vi "ex_1_main.vi"() -> ()   [LabVIEW 2020]
uses:
  <vilib>/DAQmx/read.llb/DAQmx Read (Analog 1D Wfm NChan NSamp).vi
  <vilib>/DAQmx/create/channels.llb/DAQmx Create Channel (AI-Voltage-Basic).vi
  <vilib>/DAQmx/configure/timing.llb/DAQmx Timing (Sample Clock).vi
  <vilib>/DAQmx/configure/trigger.llb/DAQmx Start Trigger (Digital Edge).vi
  <vilib>/DAQmx/miscellaneous.llb/DAQmx Fill In Error Info.vi
panel:
  out "current time 2":timestamp
  out "current time":timestamp
  out "Numeric 2":dbl
  out "Numeric":i32
  out "Waveform Graph":waveform(dbl)[](graph)
  in  "stop":bool
  # "Pomiar ciągły z 3 kanałów dowolnej (np. 6259) karty pomiarowej symulowanej w MAX dla pomiaru sygnału o częstotliwości 15kHz. Pomiar rozpoczyna się po wystąpieniu triggera na linii PFI0 wybranej karty pomiarowej."
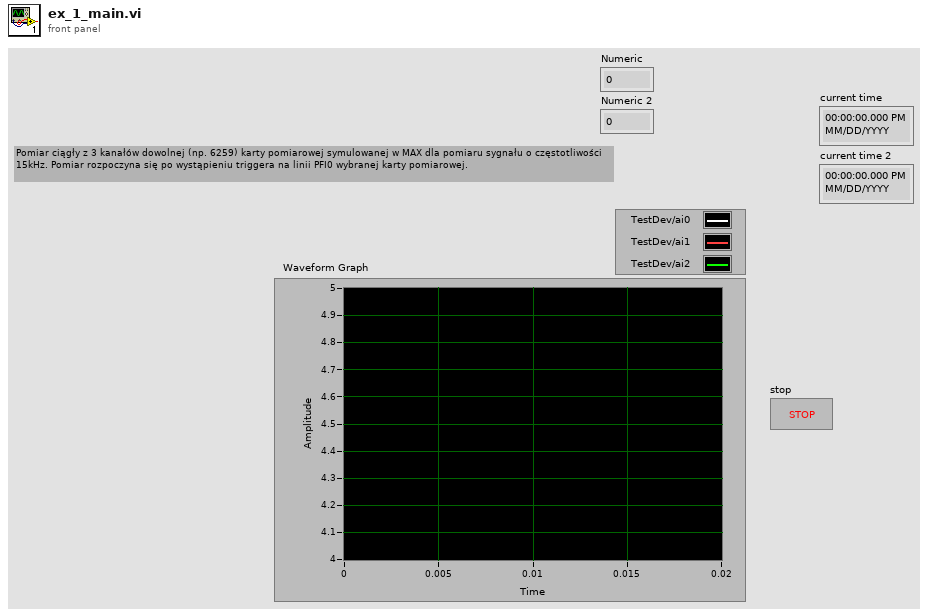
[diagram p1: front panel]
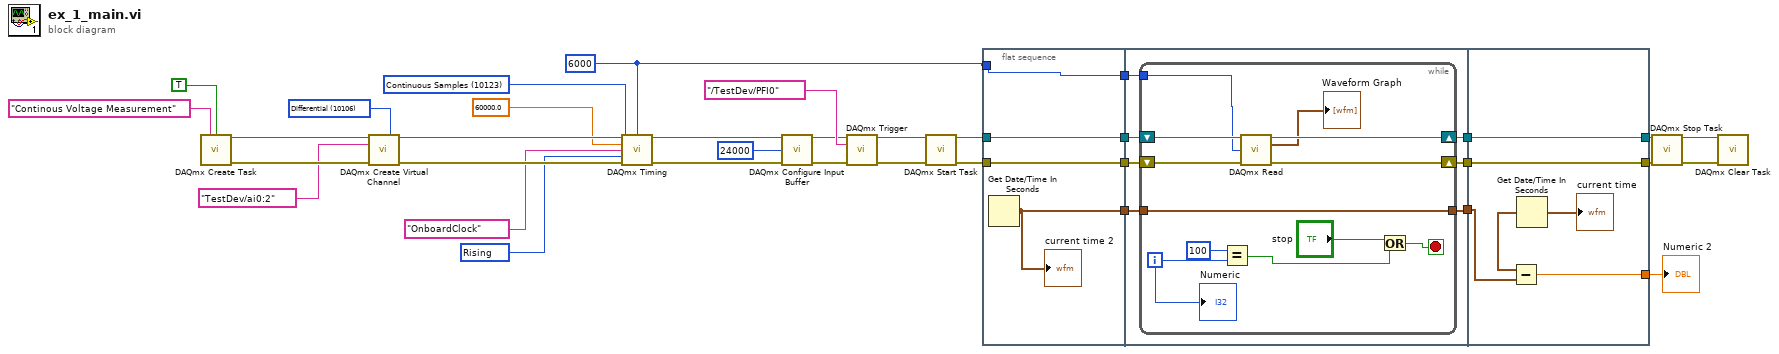
[diagram p0: block diagram]
diagram:
  w1 = 6000 ("samples per channel")
  w15 = 10106 items=["Default"=-1, "RSE"=10083, "NRSE"=10078, "Differential"=10106, "Pseudodifferential"=12529] ("input terminal configuration")
  w26 = 10280 items=["Rising"=10280, "Falling"=10171] ("active edge")
  w27 = 10123 items=["Finite Samples"=10178, "Continuous Samples"=10123, "Hardware Timed Single Point"=12522] ("sample mode")
  n1 = call <vilib>:"DAQmx Create Task.vi"("new task name"="Continous Voltage Measurement", "auto cleanup"=TRUE) -> ("task out"=w14:refnum<k21>, "error out"=w31:errorcluster)  [unwired: 12 in]
  n2 = call-poly <vilib>:"DAQmx Create Virtual Channel.vi"("task in"=w14, "input terminal configuration"=w15, "physical channels"=tag "TestDev/ai0:2", "error in"=w31) -> ("task out"=w32:refnum<k21>, "error out"=w30:errorcluster)  [unwired: 10 in]
  n3 = call-poly <vilib>:"DAQmx Timing.vi"("task/channels in"=w32, "sample mode"=w27, "samples per channel"=w1, "rate"=60000.0, "source"=tag "OnboardClock", "active edge"=w26, "error in"=w30) -> ("task out"=w22:refnum<k21>, "error out"=w21:errorcluster)  [unwired: 7 in]
  n4 = call <vilib>:"DAQmx Configure Input Buffer.vi"("task/channels in"=w22, "buffer size (in samples per channel)"=u32 24000) -> ("task out"=w13:refnum<k21>)  [unwired: 12 in, 1 out]
  n5 = call-poly <vilib>:"DAQmx Trigger.vi"("task/channels in"=w13, "source"=tag "/TestDev/PFI0", "error in"=w21) -> ("task out"=w20:refnum<k21>, "error out"=w19:errorcluster)  [unwired: 11 in]
  n6 = call <vilib>:"DAQmx Start Task.vi"("task/channels in"=w20) -> ("task out"=w11:refnum<k21>)  [unwired: 13 in, 1 out]
  n7 = flat-sequence {
    tunnel: w11 -> [w35]
    tunnel: w19 -> [w36]
    tunnel: [w36] -> w7
    tunnel: [w35] -> w6
    tunnel: [w34] -> w5
    tunnel: [w33] -> w2
    tunnel: w1 -> [w33]
    tunnel: [w42] -> w9
    tunnel: [w41] -> w8
    tunnel: w7 -> [w43]
    tunnel: w6 -> [w40]
    tunnel: w5 -> [w39]
    tunnel: [w38] -> w4
    tunnel: w2 -> [w37]
    tunnel: [w59] -> w17
    tunnel: [w60] -> w18
    tunnel: w9 -> [w60]
    tunnel: w8 -> [w59]
    tunnel: w4 -> [w56]
    tunnel: [w58] -> w3
    frame #0 {
      n8 = Get Date/Time In Seconds() -> (seconds since 1Jan1904=w34:timestamp)
      "current time 2" <- w34
    }
    frame #1 {
      n9 = while {
        shift-right: [w55] -> w42
        shift-left: w40 -> [w51]
        shift-right: [w54] -> w41
        shift-left: w43 -> [w50]
        tunnel: w39 -> [w49]
        tunnel: [w49] -> w38
        tunnel: w37 -> [w44]
        i -> [w48]
        stop <- w46 stop-if-true
        n10 = Equal?(x=100, y=w48) -> (x = y?=w45:bool)
        n11 = call-poly <vilib>:"DAQmx Read.vi"("task/channels in"=w51, "number of samples per channel"=w44, "error in"=w50) -> ("task out"=w55:refnum<k21>, "data"=→"Waveform Graph":waveform(dbl)[], "error out"=w54:errorcluster)  [unwired: 10 in]
        n12 = Or(x="stop", y=w45) -> (x .or. y?=w46:bool)
        "Numeric" <- w48
      }
    }
    frame #2 {
      n13 = Get Date/Time In Seconds() -> (seconds since 1Jan1904=w57:timestamp)
      "current time" <- w57
      n14 = Subtract(x=w57, y=w56) -> (x-y=w58:dbl)
    }
  }
  n15 = call <vilib>:"DAQmx Stop Task.vi"("task/channels in"=w18) -> ("task out"=w10:refnum<k21>)  [unwired: 13 in, 1 out]
  n16 = call <vilib>:"DAQmx Clear Task.vi"("task in"=w10, "error in"=w17) -> ()  [unwired: 13 in, 1 out]
  "Numeric 2" <- w3
